vi "PIDController.vi"(1 "e_Sum_Old":dbl, 5 "Ki":dbl, 6 "Kd":dbl, 7 "Kp":dbl, 8 "eOld":dbl, 9 "Measurement":dbl, 10 "Reference":dbl) -> (0 "u":dbl, 2 "e_Sum":dbl, 3 "e":dbl)   [LabVIEW 2019]
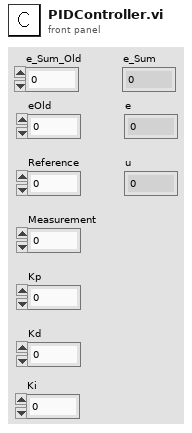
[diagram p1: front panel]
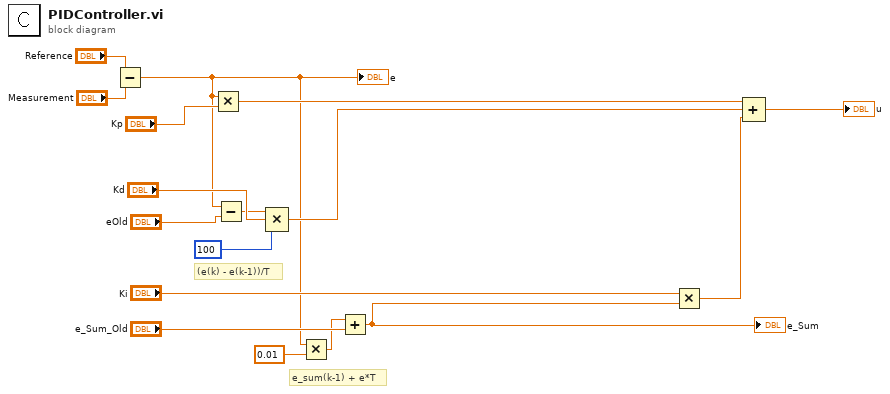
[diagram p0: block diagram]
diagram:
  # "e_sum(k-1) + e*T"
  # "(e(k) - e(k-1))/T"
  n1 = Subtract(x="Reference", y="Measurement") -> (x-y=w2:dbl)
  "e" <- w2
  n2 = Multiply(x=w2, y="Kp") -> (x*y=w12:dbl)
  n3 = Subtract(x=w2, y="eOld") -> (x-y=w14:dbl)
  n4 = Compound Arithmetic op=MULTIPLY(w14, "Kd", 100) -> (w15:dbl)
  n5 = Multiply(x=w2, y=0.01) -> (x*y=w3:dbl)
  n6 = Add(x=w3, y="e_Sum_Old") -> (x+y=w1:dbl)
  "e_Sum" <- w1
  n7 = Multiply(x="Ki", y=w1) -> (x*y=w5:dbl)
  n8 = Compound Arithmetic op=ADD(w12, w15, w5) -> (→"u":dbl)
